vi "RAM stream check.vi"() -> ()   [LabVIEW 2024]
uses:
  <vilib>/Utility/file.llb/Read Delimited Spreadsheet (DBL).vi
panel:
  in  "bitnes":enum16{"32", "64"}(ring)=enum."64"
  out "x-y":u32 format="%d (0x%x)"
  out "tot":u32
  out "pre":u32
  out "writer - osc":dbl
  out "element before zero flag, adj for buffer":u32
  out "trigger mark position":i32 format="%d (0x%x)"
  out "Write pos at trig":dbl format="%#_6f"
  out "x/y":dbl
  out "element at trig adj for buffer":u32
  out "buffer cicles":i32=8388608 format="%d (0x%x)"
  in  "buffer size":i32=67108864 format="%d (0x%x)"
  out "element at trig":u32
  in  "Pre trigger delay":u32=8192 format="%d (0x%x)"
  out "x*y":u32
  out "osc pos":u32
  out "writer pos":u32
  out "Waveform Graph 2":u64[][](graph)
  out "Difference graph":cluster{dbl, "y":dbl, i64[]}(graph)
  in  "File Path":path
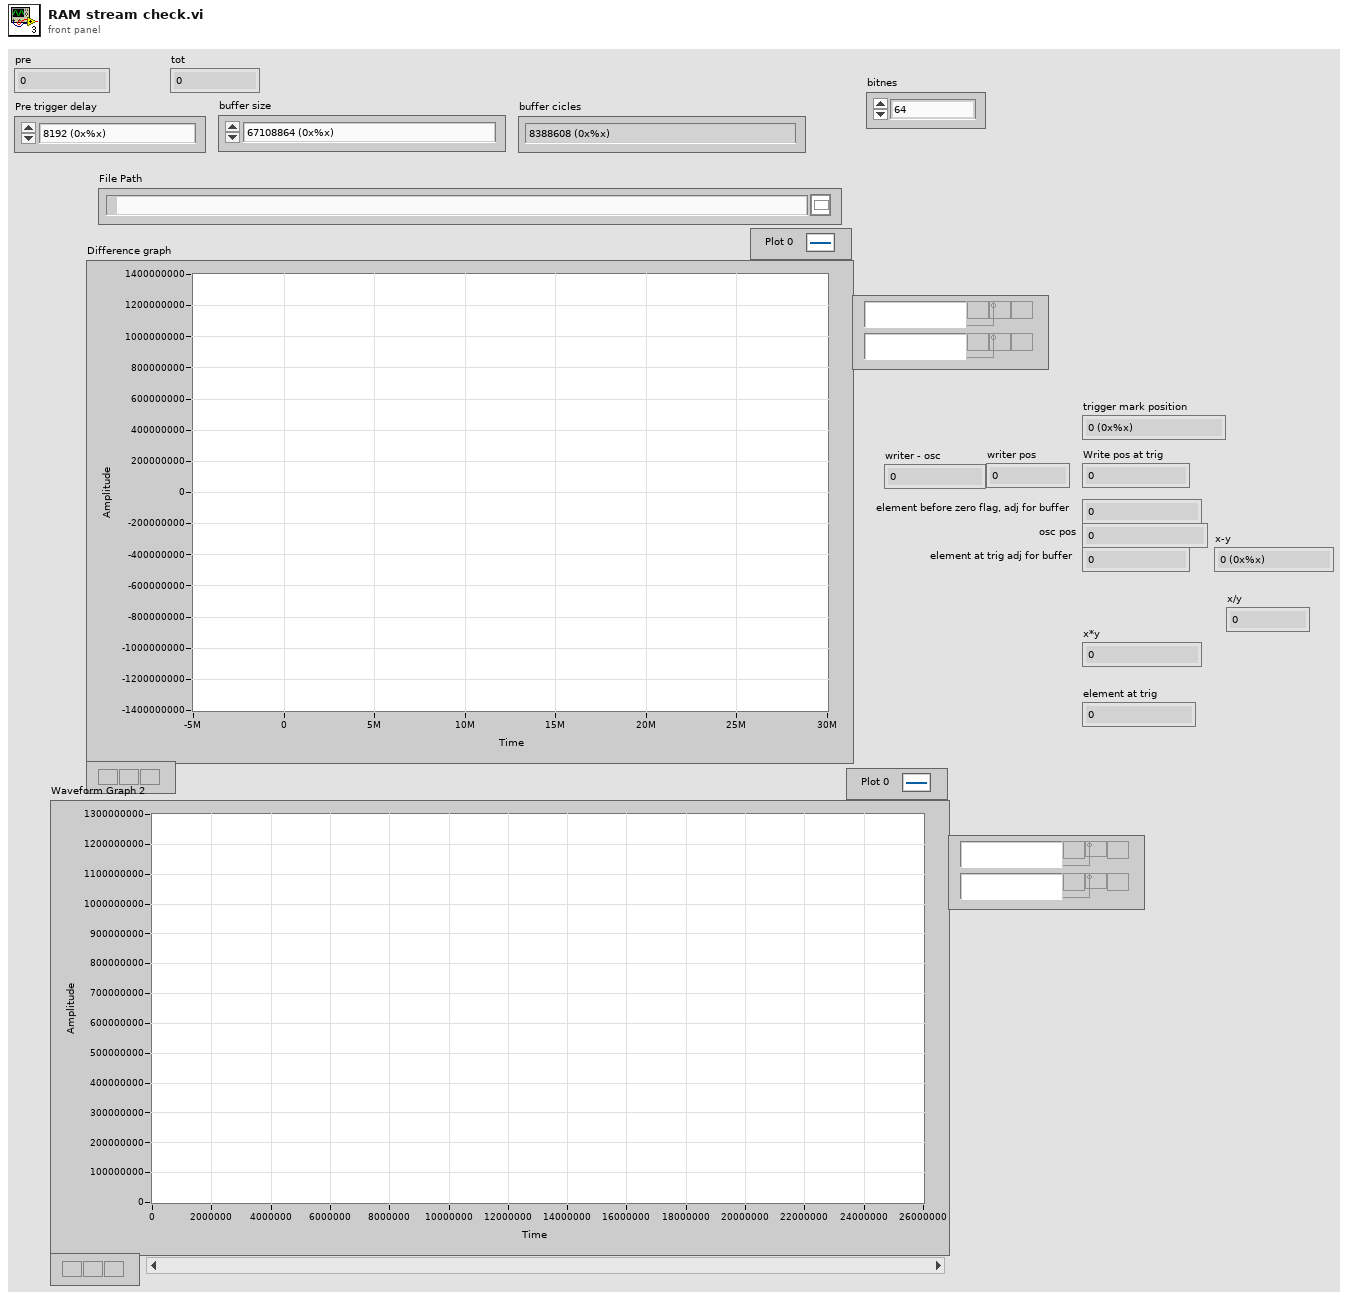
[diagram p1: front panel]
types:
  T1 = enum16{"big-endian, network order", "native, host order", "little-endian"}
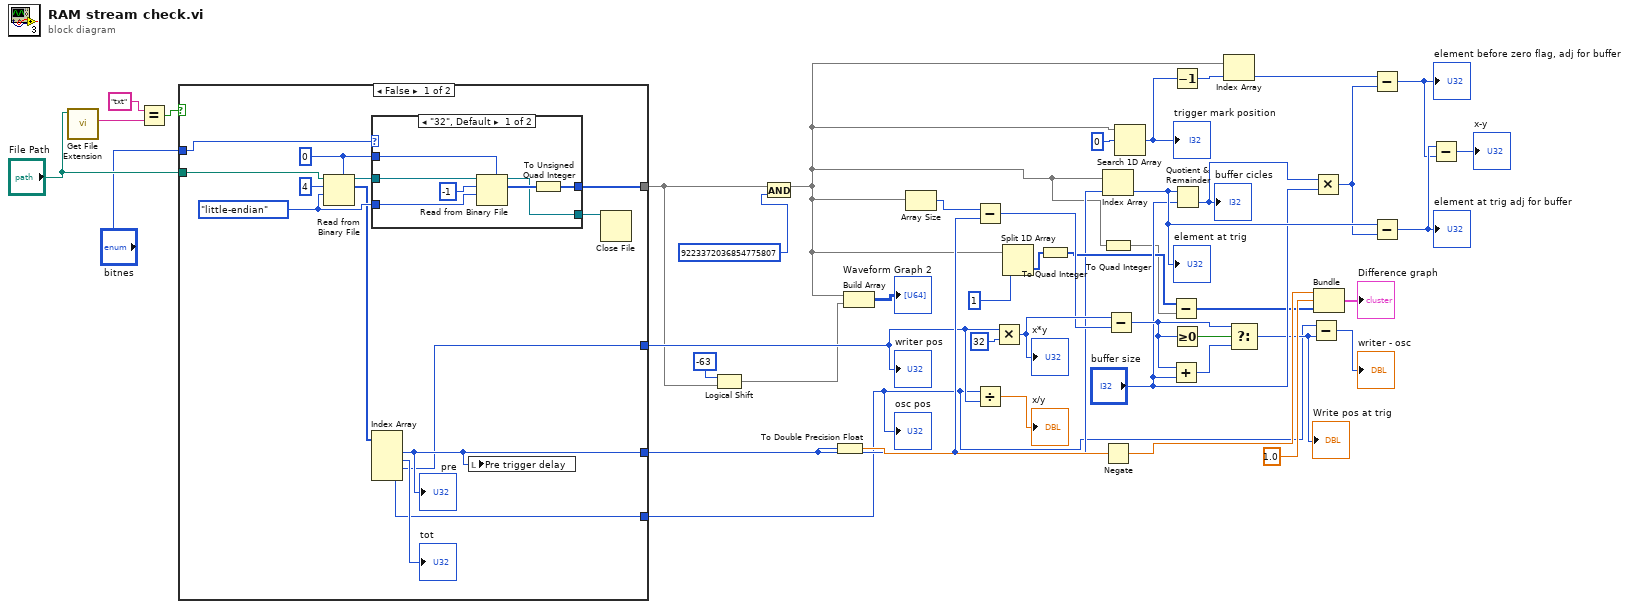
[diagram p0: block diagram]
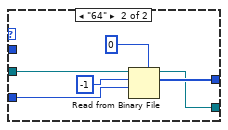
[diagram p2: hidden frame]
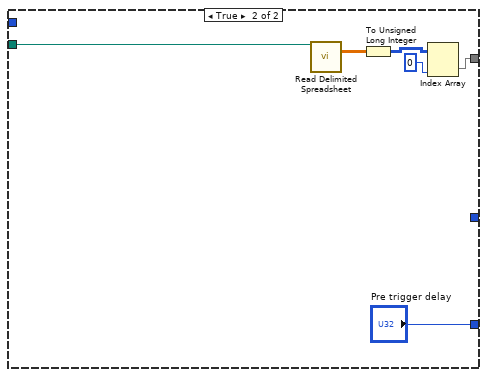
[diagram p3: hidden frame]
diagram:
  n1 = call <vilib>:"Get File Extension.vi"("file"="File Path") -> ("lowercase file extension"=w18:string)  [unwired: 6 in, 4 out]
  n2 = Equal?(x="txt", y=w18) -> (x = y?=w16:bool)
  n3 = case shown="False" w16 {
    tunnel: "File Path" -> [w57 w75]
    tunnel: [w48 w72] -> w4
    tunnel: [w54 "Pre trigger delay"] -> w15
    tunnel: "bitnes" -> [w49 _]
    tunnel: [w46 _] -> w10
    tunnel: [w45 _] -> w9
    frame False {
      w52 = T1."little-endian" ("byte order (0:big-endian, network order)")
      w50 = u32 0
      n4 = Read from Binary File(5:w50, 9:w52, 10:4 ("count (1)"), 11:w57) -> (2:w51:u32[], 3:w53:refnum<file>)  [unwired: 2 in, 2 out]
      n5 = case shown="\"32\", Default" w49 {
        tunnel: w53 -> [w64 w70]
        tunnel: w52 -> [w63 w69]
        tunnel: w50 -> [w61 _]
        tunnel: [w59 w66] -> w48
        tunnel: [w58 w65] -> w47
        frame "32", Default {
          n6 = Read from Binary File(5:w61, 9:w63, 10:-1 ("count (1)"), 11:w64) -> (2:w60:u32[], 3:w58:refnum<file>)  [unwired: 2 in, 2 out]
          n7 = To Unsigned Quad Integer(1:w60) -> (0:w59:u64[])
        }
        frame "64" {
          n8 = Read from Binary File(5:u64 0, 9:w69, 10:-1 ("count (1)"), 11:w70) -> (2:w66:u64[], 3:w65:refnum<file>)  [unwired: 2 in, 2 out]
        }
      }
      n9 = Index Array(array=w51) -> (element #1=w54:u32, element #2=→"tot":u32, element #3=w46:u32, element #4=w45:u32)  [unwired: 4 in]
      "pre" <- w54
      n10 = local write "Pre trigger delay"(w54) -> ()
      n11 = Close File(refnum=w47) -> ()  [unwired: 1 in, 2 out]
    }
    frame True {
      n12 = call-poly <vilib>:"Read Delimited Spreadsheet.vi"("file path (dialog if empty)"=w75) -> ("all rows"=w76:dbl[][])  [unwired: 9 in, 5 out]
      n13 = To Unsigned Long Integer(number=w76) -> (unsigned 32bit integer=w74:u32[][])
      n14 = Index Array(array=w74, index (col)=0 ("index (row)")) -> (element=w72:u32[])  [unwired: 1 in]
    }
  }
  "writer pos" <- w10
  "osc pos" <- w9
  n15 = Logical Shift(y=-63, x=w4) -> (x << y=w1:u64[])
  n16 = And(x=w4, y=u64 9223372036854775807) -> (x .and. y?=w6:u64[])
  n17 = To Double Precision Float(number=w15) -> (double precision float=w28:dbl)
  n18 = Build Array(w6, w1) -> (→"Waveform Graph 2":u64[][])
  n19 = Array Size(array=w6) -> (size(s)=w40:i32)
  n20 = Subtract(x=w40, y=w15) -> (x-y=w33:u32)
  n21 = Divide(x=w9, y=w10) -> (x/y=→"x/y":dbl)
  n22 = Multiply(x=w10, y=u32 32) -> (x*y=w39:u32)
  "x*y" <- w39
  n23 = Split 1D Array(array=w6, index=1) -> (second subarray=w8:u64[])  [unwired: 1 out]
  n24 = To Quad Integer(1:w8) -> (0:w21:i64[])
  n25 = Index Array(array=w6, index=w15) -> (element=w43:u64)
  "element at trig" <- w43
  n26 = To Quad Integer(1:w6) -> (0:w20:i64[])
  n27 = Negate(x=w28) -> (-x=w27:dbl)
  n28 = Subtract(x=w39, y=w33) -> (x-y=w31:u32)
  n29 = Search 1D Array(1D array=w6, element=u32 0) -> (index of element=w37:i32)  [unwired: 1 in]
  "trigger mark position" <- w37
  n30 = Subtract(x=w21, y=w20) -> (x-y=w25:i64[])
  n31 = Add(x=w31, y="buffer size") -> (x+y=w29:u32)
  n32 = Decrement(x=w37) -> (x-1=w36:i32)
  n33 = Greater Or Equal To 0?(x=w31) -> (x >= 0?=w32:bool)
  n34 = Quotient & Remainder(x=w43, y="buffer size") -> (floor(x/y)=w42:u64)  [unwired: 1 out]
  "buffer cicles" <- w42
  n35 = Index Array(array=w6, index=w36) -> (element=w35:u64)
  n36 = Select(t=w31, s=w32, f=w29) -> (s? t:f=w23:u32)
  "Write pos at trig" <- w23
  n37 = Subtract(x=w9, y=w23) -> (x-y=→"writer - osc":u32)
  n38 = Multiply(x=w42, y="buffer size") -> (x*y=w34:u64)
  n39 = Bundle(w27, "y"=1.0, w25) -> (→"Difference graph":cluster{dbl, "y":dbl, i64[]})  [unwired: 1 in]
  n40 = Subtract(x=w35, y=w34) -> (x-y=w13:u64)
  "element before zero flag, adj for buffer" <- w13
  n41 = Subtract(x=w43, y=w34) -> (x-y=w14:u64)
  "element at trig adj for buffer" <- w14
  n42 = Subtract(x=w14, y=w13) -> (x-y=→"x-y":u64)
